vi "GetInstrMenuPan.vi"(8 "error in (no error)":errorcluster caption="entrée d'erreur (pas d'erreur)", 10 "référence de menu":refnum<k9>, 11 "Experiment en entrée":refnum<class "Experiment.lvclass"> caption="DNL_LabVIEW Object in") -> (0 "error out":errorcluster caption="sortie d'erreur", 3 "Experiment en sortie":refnum<class "Experiment.lvclass"> caption="DNL_LabVIEW Object out")   [LabVIEW 2019, in "Experiment.lvclass"]
uses:
  Experiment.lvclass
  Experiment.lvclass/Experiment.ctl
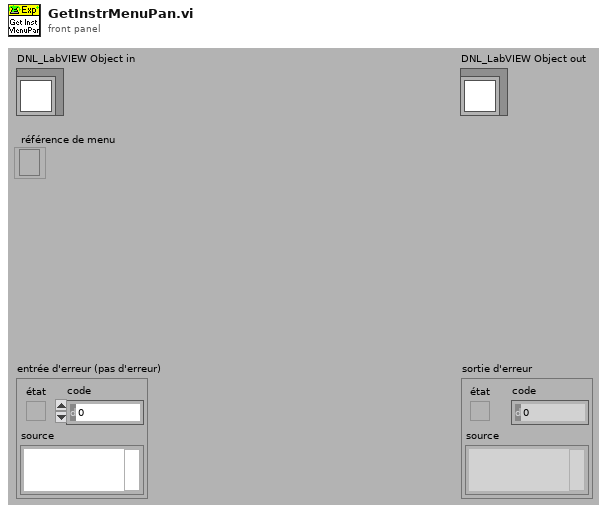
[diagram p1: front panel]
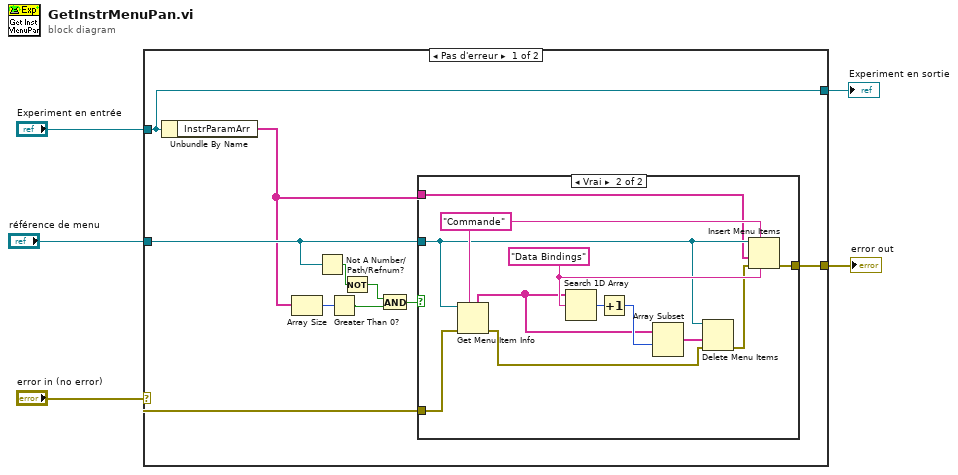
[diagram p0: block diagram]
diagram:
  n1 = case shown="Pas d'erreur" "error in (no error)" {
    selector: "error in (no error)" -> [w6 w30]
    tunnel: [w15 w30] -> w4
    tunnel: [w7 w29] -> w2
    tunnel: "Experiment en entrée" -> [w7 w29]
    tunnel: "référence de menu" -> [w12 _]
    frame No Error {
      n2 = Unbundle By Name(w7) -> ("InstrParamArr"=w10:string[])
      n3 = Array Size(array=w10) -> (size(s)=w9:i32)
      n4 = Not A Number/Path/Refnum?(number/path/refnum=w12) -> (NaN/Path/Refnum?=w13:bool)
      n5 = Greater Than 0?(x=w9) -> (x > 0?=w8:bool)
      n6 = Not(x=w13) -> (.not. x?=w11:bool)
      n7 = And(x=w11, y=w8) -> (x .and. y?=w14:bool)
      n8 = case shown="Vrai" w14 {
        tunnel: w12 -> [_ w18]
        tunnel: w6 -> [w16 w20]
        tunnel: [w16 w19] -> w15
        tunnel: w10 -> [_ w17]
        frame False {
        }
        frame True {
          w27 = "Data Bindings" ("élément suivant")
          w23 = "Commande" ("tag de menu")
          n9 = Get Menu Item Info(7:w23, 8:w20, 11:w18) -> (0:w22:errorcluster, 5:w24:string[])  [unwired: 5 out]
          n10 = Search 1D Array(1D array=w24, element=w27) -> (index of element=w25:i32)  [unwired: 1 in]
          n11 = Increment(x=w25) -> (x+1=w28:i32)
          n12 = Array Subset(array=w24, index=w28) -> (w26:string[])  [unwired: 1 in]
          n13 = Delete Menu Items(6:w22, 7:w26, 9:w18) -> (0:w21:errorcluster)  [unwired: 1 in, 1 out]
          n14 = Insert Menu Items(4:w27, 5:w23, 6:w21, 7:w17, 9:w18) -> (0:w19:errorcluster)  [unwired: 1 in, 2 out]
        }
      }
    }
    frame Error {
    }
  }
  "error out" <- w4
  "Experiment en sortie" <- w2
